vi "Heap Exchange.vi"(8 "error in (no error)":errorcluster, 9 "Results Heap":variant, 10 "tdms file":refnum<k34>, 11 "Mag Lab Result in":refnum<class "Mag Lab Result.lvclass">) -> (0 "error out":errorcluster, 1 "Results Heap out":variant, 2 "tdms file out":refnum<k34>, 3 "Mag Lab Result out":refnum<class "Mag Lab Result.lvclass">)   [LabVIEW 2015, in "Mag Lab Result.lvclass"]
uses:
  Mag Lab Result.lvclass
  Mag Lab Result.lvclass/Mag Lab Result.ctl
  Payload/Payload.lvclass/Payload.ctl
  Payload/Payload.lvclass
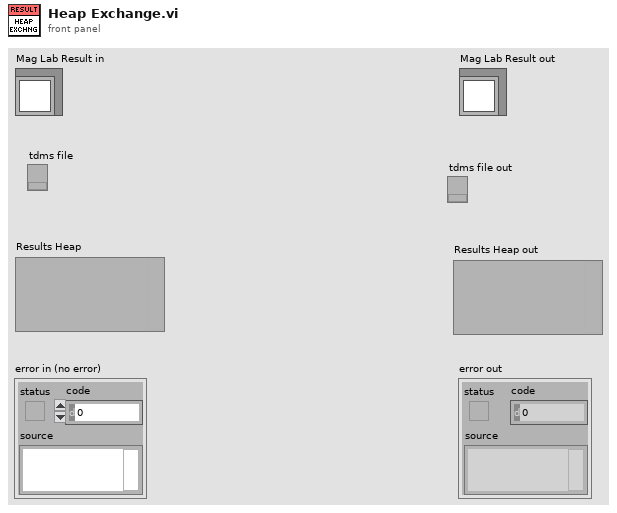
[diagram p1: front panel]
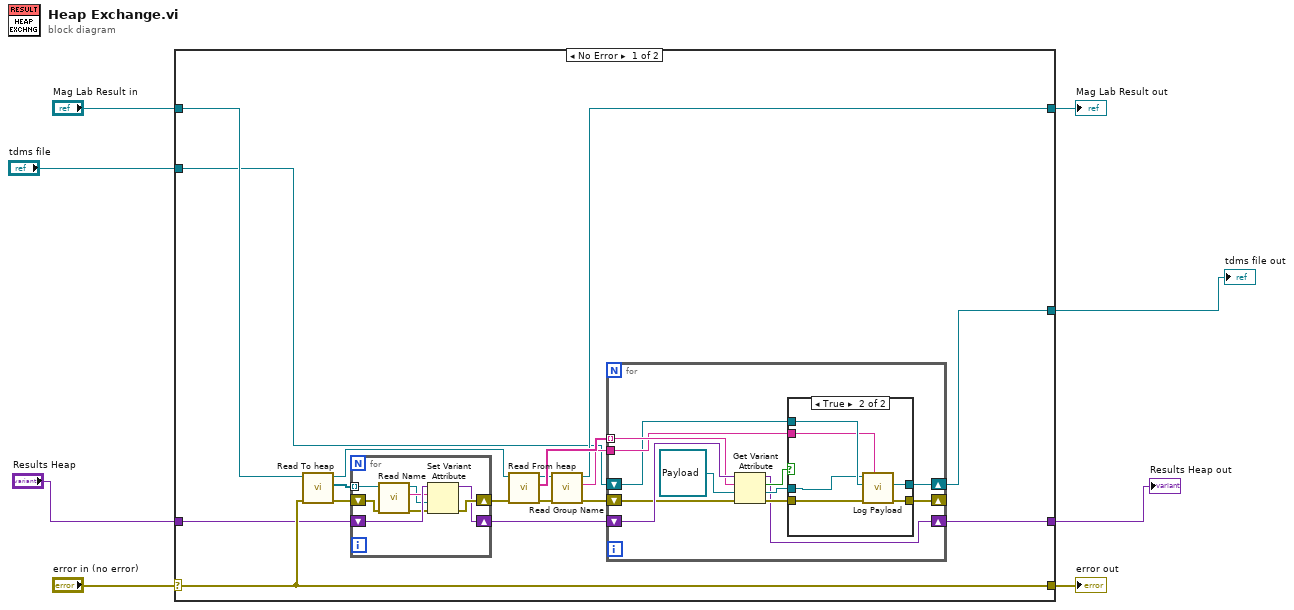
[diagram p0: block diagram]
diagram:
  n1 = case shown="No Error" "error in (no error)" {
    selector: "error in (no error)" -> [w14 w57]
    tunnel: [w14 w57] -> w7
    tunnel: [w11 w56] -> w5
    tunnel: "Mag Lab Result in" -> [w15 w56]
    tunnel: [w13 w54] -> w4
    tunnel: "Results Heap" -> [w12 w54]
    tunnel: "tdms file" -> [w10 w55]
    tunnel: [w9 w55] -> w1
    frame No Error {
      n2 = call "Read To heap.vi"("error in (no error)"=w14, "Mag Lab Result in"=w15) -> ("error out"=w24:errorcluster, "To heap"=w25:refnum<class "Payload.lvclass">[], "Mag Lab Result out"=w21:refnum<class "Mag Lab Result.lvclass">)  [unwired: 7 in]
      n3 = for {
        tunnel: w25 -> [w53] mode=indexing
        shift-right: [w47] -> w23
        shift-left: w24 -> [w52]
        shift-right: [w46] -> w20
        shift-left: w12 -> [w51]
        n4 = call "Read Name.vi"("error in (no error)"=w52, "Payload in"=w53) -> ("error out"=w50:errorcluster, "Name"=w49:string, "Payload out"=w48:refnum<class "Payload.lvclass">)  [unwired: 7 in]
        n5 = Set Variant Attribute(Variant=w51, name=w49, value=w48, error in=w50) -> (Variant out=w46:variant, error out=w47:errorcluster)  [unwired: 1 out]
      }
      n6 = call "Read From heap.vi"("error in (no error)"=w23, "Mag Lab Result in"=w21) -> ("error out"=w18:errorcluster, "From heap"=w22:string[], "Mag Lab Result out"=w19:refnum<class "Mag Lab Result.lvclass">)  [unwired: 7 in]
      n7 = call "Read Group Name.vi"("error in (no error)"=w18, "Mag Lab Result in"=w19) -> ("error out"=w17:errorcluster, "Group Name"=w16:string, "Mag Lab Result out"=w11:refnum<class "Mag Lab Result.lvclass">)  [unwired: 7 in]
      n8 = for {
        shift-right: [w27] -> _
        shift-left: w17 -> [w35]
        shift-right: [w26] -> w13
        shift-left: w20 -> [w37]
        tunnel: w22 -> [w36] mode=indexing
        tunnel: w16 -> [w31]
        shift-right: [w28] -> w9
        shift-left: w10 -> [w29]
        n9 = Get Variant Attribute(Variant=w37, name=w36, default value (empty Variant)=refnum<class "Payload.lvclass"> refnum ("Mag Lab Result out"), error in=w35) -> (duplicate Variant=w26:variant, found=w33:bool, value=w30:refnum<class "Payload.lvclass">, error out=w32:errorcluster)
        n10 = case shown="True" w33 {
          tunnel: w32 -> [w38 w42]
          tunnel: w31 -> [_ w40]
          tunnel: w30 -> [_ w41]
          tunnel: w29 -> [w39 w45]
          tunnel: [w39 w44] -> w28
          tunnel: [w38 w43] -> w27
          frame False {
          }
          frame True {
            n11 = call-dynamic "Log Payload.vi"("Group Name"=w40, "error in (no error)"=w42, "tdms file"=w45, "Payload in"=w41) -> ("error out"=w43:errorcluster, "tdms file out"=w44:refnum<k34>)  [unwired: 5 in, 1 out]
          }
        }
      }
    }
    frame Error {
    }
  }
  "error out" <- w7
  "Mag Lab Result out" <- w5
  "Results Heap out" <- w4
  "tdms file out" <- w1
